vi "saveSettings.vi"(8 "error in (no error)":errorcluster, 10 "Path":path, 11 "SettingsManager in":refnum<class "SettingsManager.lvclass">) -> (0 "error out":errorcluster, 3 "SettingsManager out":refnum<class "SettingsManager.lvclass">)   [LabVIEW 2011, in "Tools.lvlib" / "Settings.lvlib" / "SettingsManager.lvclass"]
uses:
  SettingsManager.lvclass
  SettingsManager.lvclass/SettingsManager.ctl
  xmlNode/xmlNode.lvclass
  XmlParser.lvclass
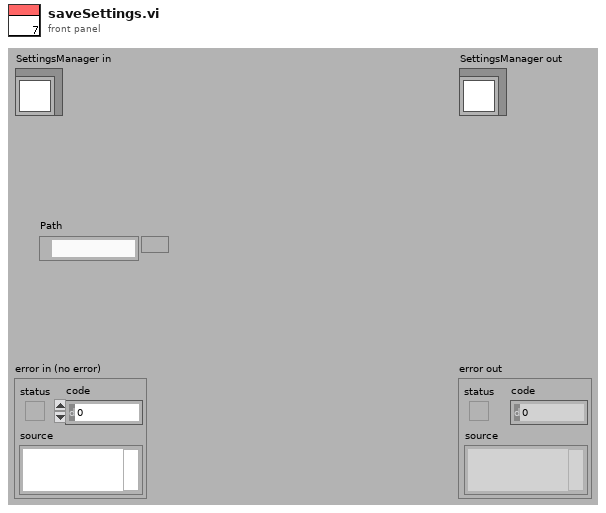
[diagram p1: front panel]
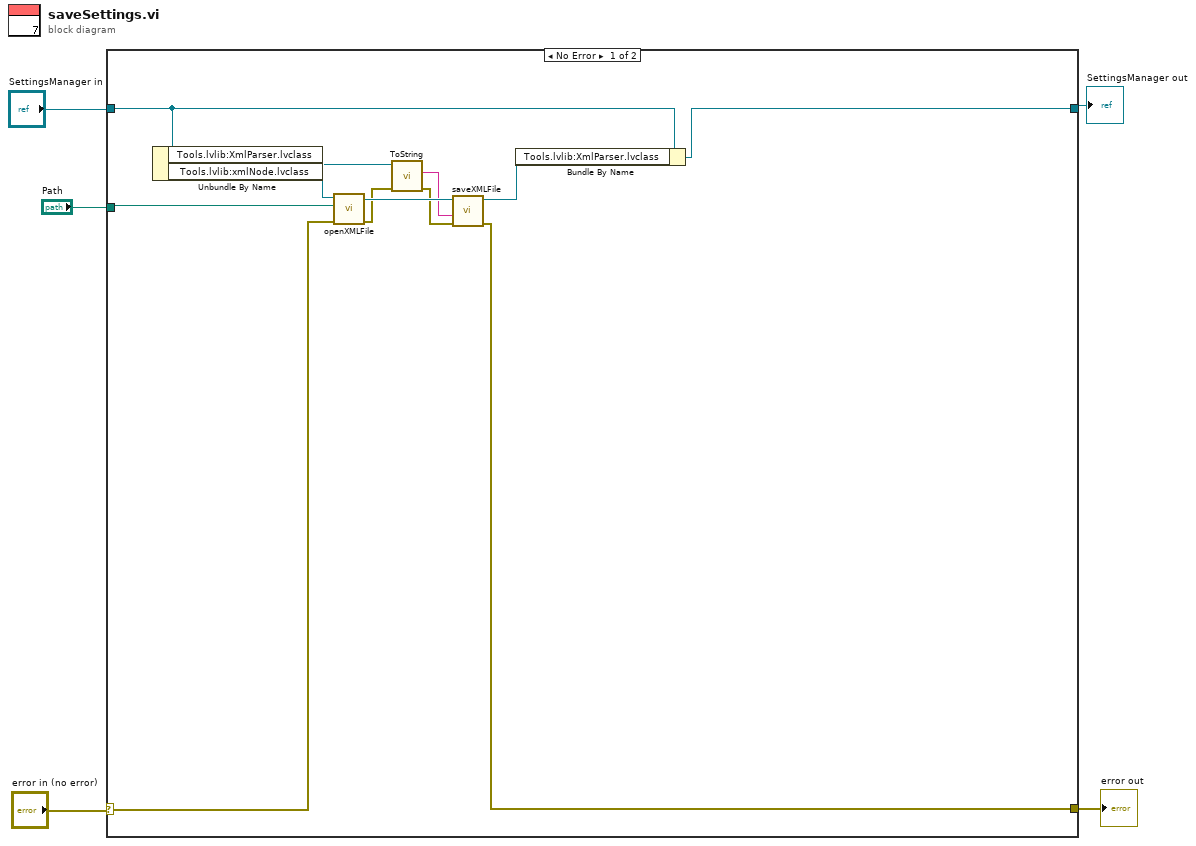
[diagram p0: block diagram]
diagram:
  n1 = case shown="No Error" "error in (no error)" {
    selector: "error in (no error)" -> [w15 w19]
    tunnel: [w12 w19] -> w4
    tunnel: [w10 w18] -> w2
    tunnel: "SettingsManager in" -> [w11 w18]
    tunnel: "Path" -> [w16 _]
    frame No Error {
      n2 = Unbundle By Name(w11) -> ("Tools.lvlib:XmlParser.lvclass"=w17:refnum<class "XmlParser.lvclass">, "Tools.lvlib:xmlNode.lvclass"=w9:refnum<class "xmlNode.lvclass">)
      n3 = call "openXMLFile.vi"("error in (no error)"=w15, "Path"=w16, "XmlParser in"=w17) -> ("error out"=w8:errorcluster, "XmlParser out"=w14:refnum<class "XmlParser.lvclass">)  [unwired: 6 in, 1 out]
      n4 = call-dynamic "ToString.vi"("error in (no error)"=w8, "xmlNode in"=w9) -> ("error out"=w7:errorcluster, "xml"=w6:string)  [unwired: 7 in, 1 out]
      n5 = call-dynamic "saveXMLFile.vi"("error in (no error)"=w7, "xmlString"=w6, "XmlParser in"=w14) -> ("error out"=w12:errorcluster, "XmlParser out"=w13:refnum<class "XmlParser.lvclass">)  [unwired: 7 in]
      n6 = Bundle By Name(cluster=w11, "Tools.lvlib:XmlParser.lvclass"=w13) -> (w10:refnum<class "SettingsManager.lvclass">)
    }
    frame Error {
    }
  }
  "error out" <- w4
  "SettingsManager out" <- w2
